vi "Use case.vi"() -> ()   [LabVIEW 2024]
uses:
  controls/SN_length.ctl
  controls/SN_parse_mode.ctl
  controls/SN_device_type.ctl
  controls/SN Data.ctl
  controls/SN_device_type_out.ctl
  libraries/API-Config-Files-Management/API Config Files Management.lvlib
panel:
  out "SN Data":T1
  out "error out":errorcluster
  in  "Device Type":T3
  in  "Parse mode":T4
  in  "Length range":T5
  in  "Serial Number in":string
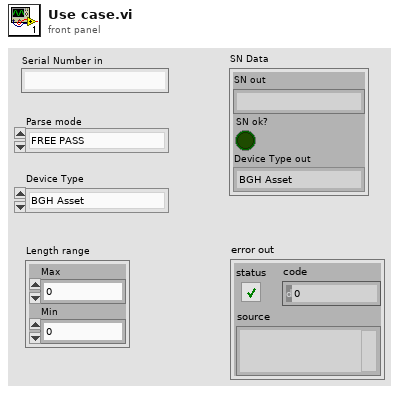
[diagram p1: front panel]
types:
  T1 = typedef "SN Data.ctl" = cluster{"SN out":string, "SN ok?":bool, "Device Type out":T2}
  T2 = typedef "SN_device_type_out.ctl" = enum16{"BGH Asset", "BGH Product", "SAMSUNG Product", "GENERIC Product", "No Product", ""}
  T3 = typedef "SN_device_type.ctl" = enum16{"BGH Asset", "BGH Product", "SAMSUNG Product"}
  T4 = typedef "SN_parse_mode.ctl" = enum16{"FREE PASS", "LENGTH BASED", "REGEX BASED", "AUTO"}
  T5 = typedef "SN_length.ctl" = cluster{"Max":i32, "Min":i32}
  T6 = typedef "NI_LVConfig.lvlib/Config Data RefNum.ctl" = refnum<k1>
  T7 = typedef "config data.ctl" = cluster{"sections":string[][], "key names":string[], "values":string[]}
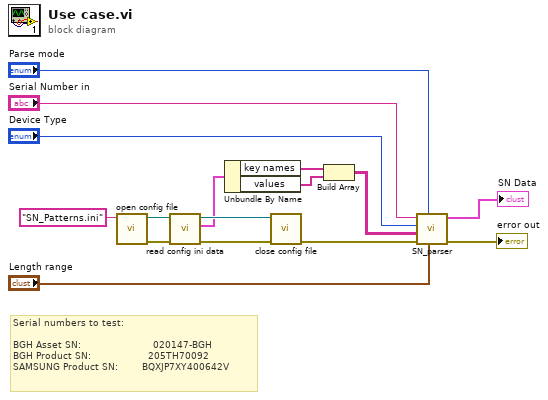
[diagram p0: block diagram]
diagram:
  # "Serial numbers to test: \n\nBGH Asset SN:                        020147-BGH\nBGH Product SN:                   205TH70092\nSAMSUNG Product SN:        BQXJP7XY400642V"
  n1 = call "open config file.vi"("file name"="SN_Patterns.ini") -> ("error out"=w16:errorcluster, "Refnum out"=w14:T6)  [unwired: 8 in, 1 out]
  n2 = call "read config ini data.vi"("error in (no error)"=w16, "Refnum in"=w14) -> ("error out"=w15:errorcluster, "data out"=w11:T7, "Refnum out"=w13:T6)  [unwired: 7 in]
  n3 = Unbundle By Name(w11) -> ("key names"=w10:string[], "values"=w9:string[])
  n4 = call "close config file.vi"("error in (no error)"=w15, "Refnum in"=w13) -> ("error out"=w3:errorcluster)  [unwired: 9 in]
  n5 = Build Array(w10, w9) -> (w8:string[][])
  n6 = call "SN_parser.vi"("Length range"="Length range", "Parse mode"="Parse mode", "error in (no error)"=w3, "Regex"=w8, "Device Type"="Device Type", "SN in"="Serial Number in") -> ("error out"=→"error out":errorcluster, "SN Data"=→"SN Data":T1)  [unwired: 4 in]
